vi "ClearAnnotationsOnTimingPlot.vi"(11 "Cluster in":refnum<vi>) -> ()   [LabVIEW 2013]
uses:
  <vilib>/Utility/miscctls.llb/LVAnnotationListTypeDef.ctl
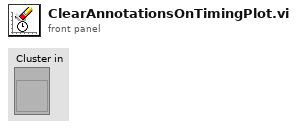
[diagram p1: front panel]
types:
  T1 = typedef "LVAnnotationListTypeDef.ctl" = cluster{"Name":string, "Color":u32, "Style":u8, "Point Style":u8, "Name Visible":bool, "Allow Drag":bool, "Annotation Mode":u32, "Plot":i32, "Index":i32, "Position":cluster{"X":dbl, "Y":dbl}, "X Scale":u32, "Y Scale":u32, "Show Arrow":bool, "Lock Name":bool, "Plot Area":i32, "Label Offset":cluster{"X":dbl, "Y":dbl}}[]
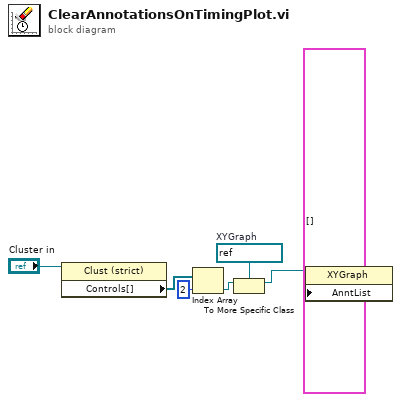
[diagram p0: block diagram]
diagram:
  w5 = refnum<vi> refnum  # XYGraph
  n1 = property class="Clust (strict)"(reference="Cluster in") -> ("Controls[]"=w2:refnum<vi>[])  [unwired: 1 in, 2 out]
  n2 = Index Array(array=w2, index=2) -> (element=w4:refnum<vi>)
  n3 = To More Specific Class(target class=w5, reference=w4) -> (specific class reference=w6:refnum<vi>)  [unwired: 1 in, 1 out]
  n4 = property class="XYGraph"(reference=w6, "AnntList"=T1 [] ("Annotation List")) -> ()  [unwired: 1 in, 2 out]
